vi "PRIME Detector Open Port Refs.vi"(8 "error in (no error)":errorcluster, 11 "Settings":T1={"Machine"="192.168.121.11", "Password"="", "FITS File Path"="", "Port"=44444, "Header Path"="", "Name"=""}) -> (0 "error out":errorcluster, 3 "Connect Refs":refnum<k5>[](array[refnum]))   [LabVIEW 2021, in "PRIME Detector.lvclass"]
uses:
  PRIME Detector.lvclass
  RIMAS Detector Server Config.ctl
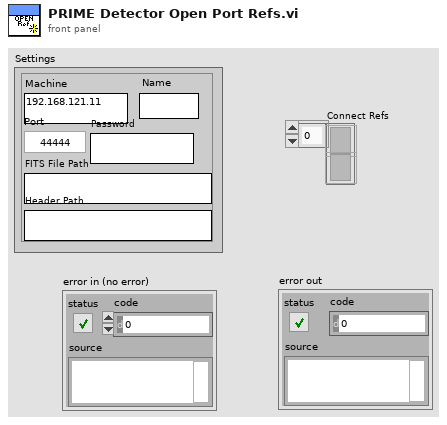
[diagram p1: front panel]
types:
  T1 = typedef "RIMAS Detector Server Config.ctl" = cluster{"Machine":string, "Password":string, "FITS File Path":string, "Port":u16, "Header Path":string, "Name":string}
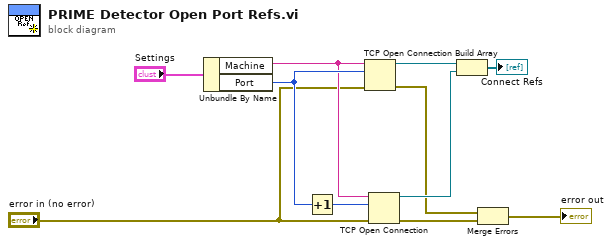
[diagram p0: block diagram]
diagram:
  n1 = Unbundle By Name("Settings") -> ("Machine"=w9:string, "Port"=w10:u16)
  n2 = Increment(x=w10) -> (x+1=w2:u16)
  n3 = TCP Open Connection(address=w9, remote port or service name=w10, error in (no error)="error in (no error)") -> (connection ID=w8:refnum<k5>, error out=w5:errorcluster)  [unwired: 2 in]
  n4 = TCP Open Connection(address=w9, remote port or service name=w2, error in (no error)="error in (no error)") -> (connection ID=w7:refnum<k5>, error out=w1:errorcluster)  [unwired: 2 in]
  n5 = Build Array(w8, w7) -> (→"Connect Refs":refnum<k5>[])
  n6 = Merge Errors(w5, w1) -> (→"error out":errorcluster)
